vi "DAQ Message Loop.vi"(8 "error in (no error)":errorcluster, 11 "Message Queues":T1) -> (0 "error out":errorcluster)   [LabVIEW 2018, in "DAQ.lvlib"]
doc: "Message loop for handling messages pertaining to the acquisition of data from the hardware."
uses:
  DAQ/DAQ.lvlib
  Main/Main Queue Cluster.ctl
  support/Message Queue/Message Cluster.ctl
  Acquisition State.ctl
  Hardware Configuration.ctl
  Task Cluster.ctl
  controls/Queue and Message Cluster.ctl
  support/Message Queue/Enqueue Message (Single).vi
  support/Message Queue/Message Queue.lvlib
  DAQ/DAQ Write Folder/DAQ/DAQ Write.lvlib
  Acquisition Settings Dialog.vi
  support/Command Log VIs/Command Logging.lvlib
  Report Generation/Report Generation.lvlib
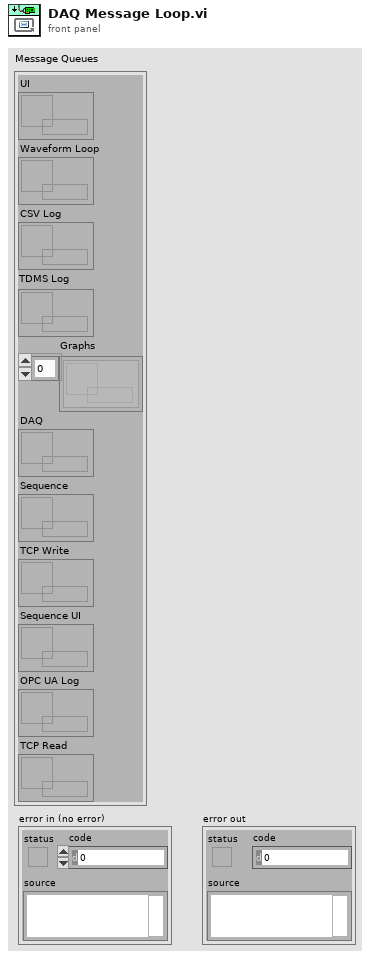
[diagram p1: front panel]
types:
  T1 = typedef "Main Queue Cluster.ctl" = cluster{"UI":refnum<queue>, "Waveform Loop":refnum<queue>, "CSV Log":refnum<queue>, "TDMS Log":refnum<queue>, "Graphs":refnum<queue>[], "DAQ":refnum<queue>, "Sequence":refnum<queue>, "TCP Write":refnum<queue>, "Sequence UI":refnum<queue>, "OPC UA Log":refnum<queue>, "TCP Read":refnum<queue>}
  T2 = typedef "DAQ.lvlib/Hardware Configuration.ctl" = cluster{"Tasks Array":T3[]}
  T3 = typedef "Task Cluster.ctl" = cluster{"DAQmx Task":refnum<k21>, "Read-Write Radio":enum32{"Read", "Write"}}
  T4 = typedef "DAQ.lvlib/DAQ Write.lvlib/Acquisition State.ctl" = enum16{"Idle", "Acquiring"}
  T5 = typedef "Queue and Message Cluster.ctl" = cluster{"return Message Queue":refnum<queue>, "Message":string, "Variant":variant}
  T6 = cluster{"Name":string, "Alarm Time":timestamp}[][]
  T7 = typedef "Message Queue.lvlib/Message Cluster.ctl" = cluster{"Message":string, "Message Data":variant}
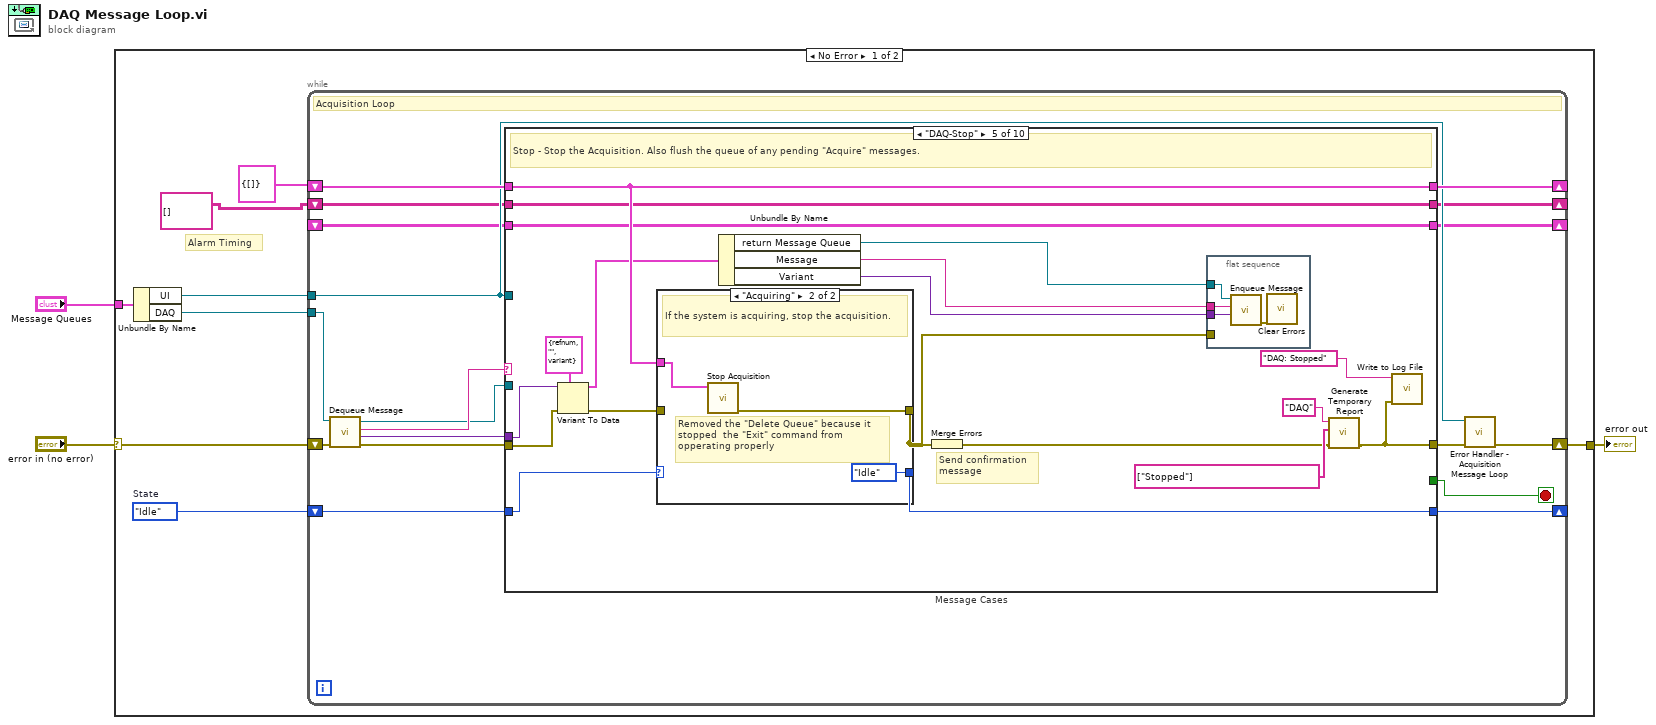
[diagram p0: block diagram]
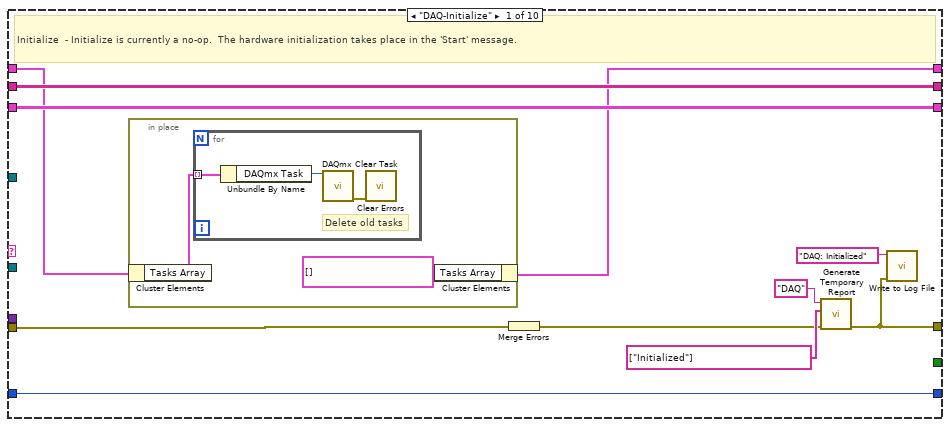
[diagram p2: hidden frame]
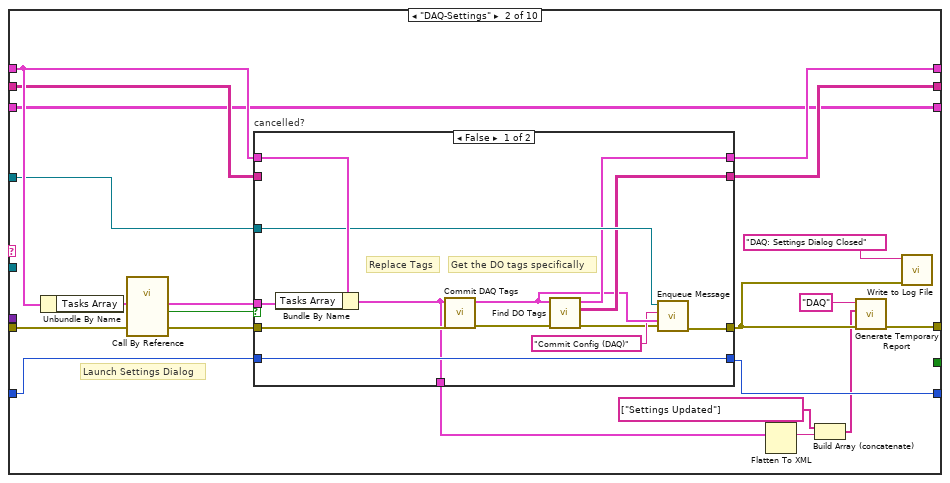
[diagram p3: hidden frame]
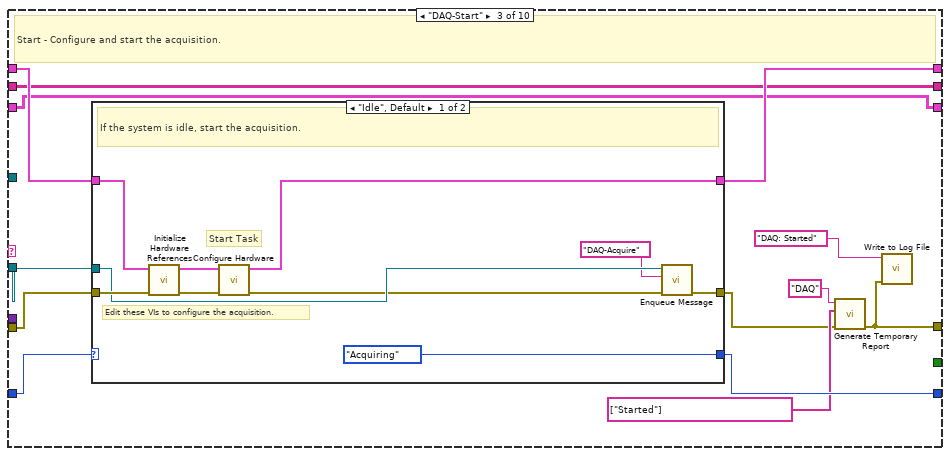
[diagram p5: hidden frame]
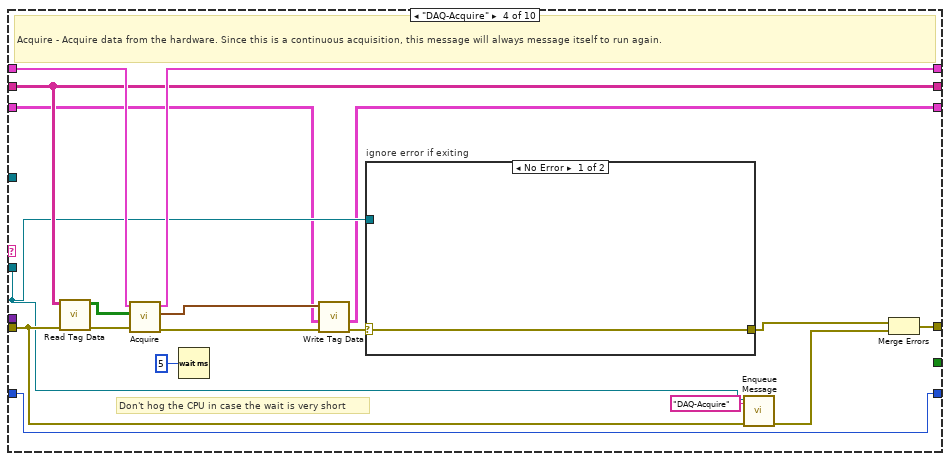
[diagram p7: hidden frame]
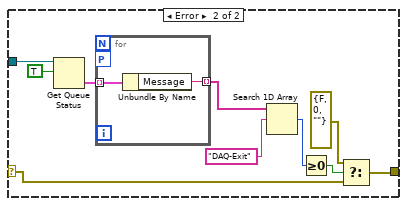
[diagram p8: hidden frame]
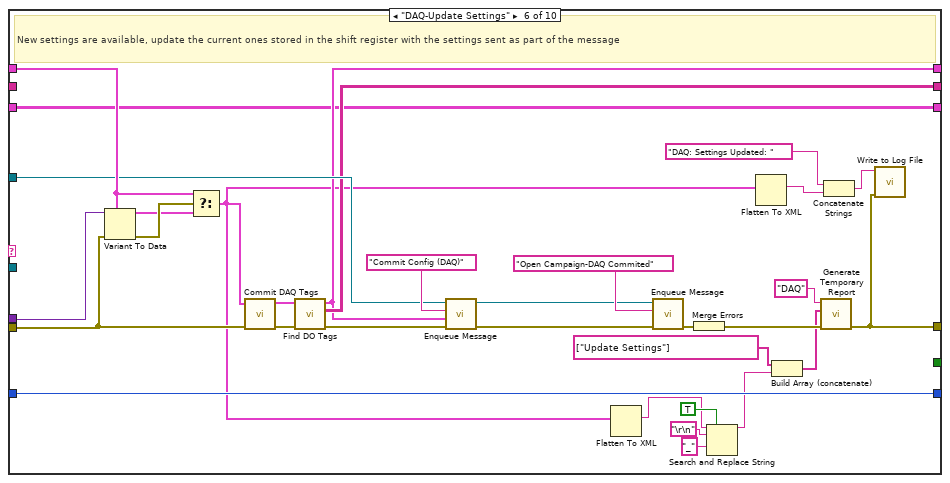
[diagram p10: hidden frame]
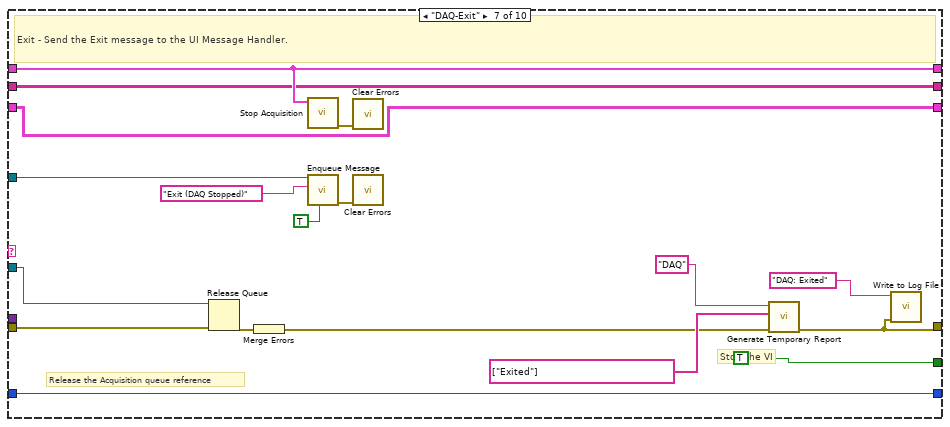
[diagram p11: hidden frame]
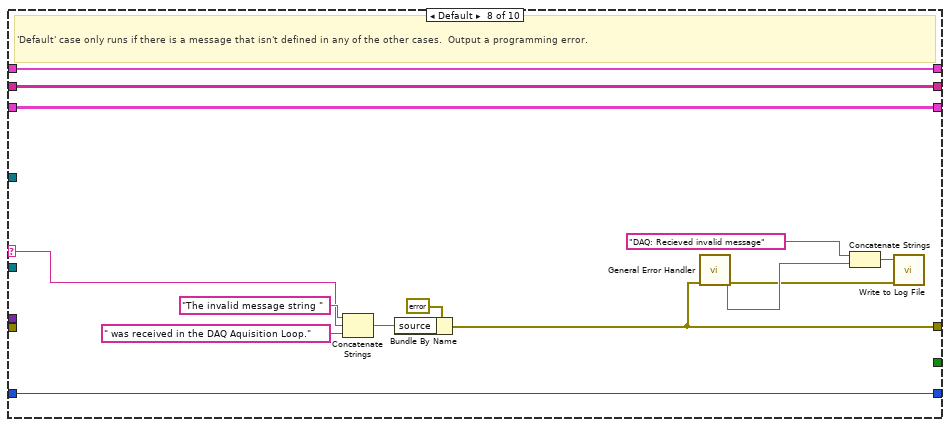
[diagram p12: hidden frame]
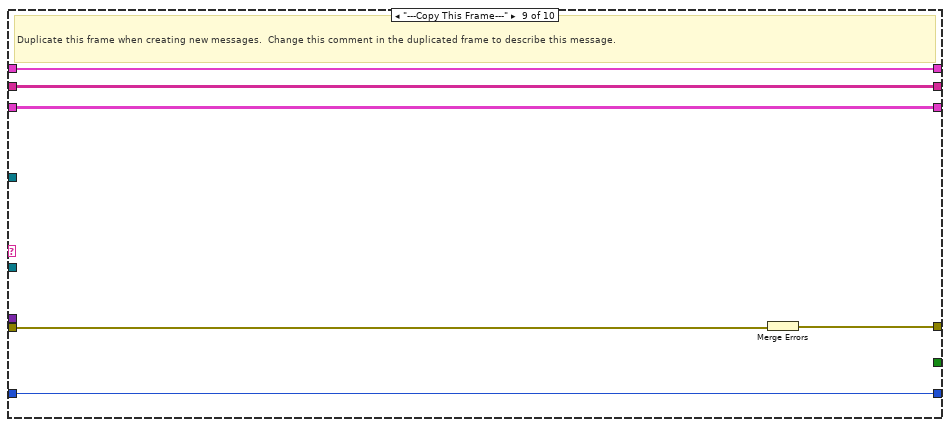
[diagram p13: hidden frame]
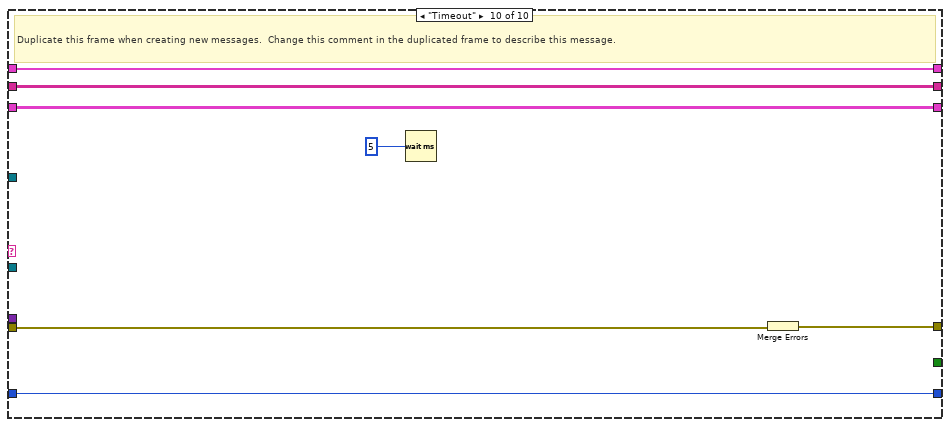
[diagram p14: hidden frame]
diagram:
  n1 = case shown="No Error" "error in (no error)" {
    selector: "error in (no error)" -> [w8 w246]
    tunnel: "Message Queues" -> [w11 _]
    tunnel: [w9 w246] -> w2
    frame No Error {
      w6 = Acquisition_State."Idle"  # State
      # "Alarm Timing"
      n2 = Unbundle By Name(w11) -> ("UI"=w7:refnum<queue>, "DAQ"=w10:refnum<queue>)
      n3 = while {
        tunnel: w10 -> [w23]
        shift-right: [w28] -> _
        shift-left: T2 {"Tasks Array"=[]} ("Data Cluster") -> [w29]
        shift-right: [w21] -> w9
        shift-left: w8 -> [w26]
        tunnel: w7 -> [w20]
        shift-right: [w18] -> _
        shift-left: w6 -> [w19]
        shift-right: [w17] -> _
        shift-left: string[][] [] ("Task D-O Channels") -> [w16]
        shift-right: [w13] -> _
        shift-left: _ -> [w12]
        stop <- w27 stop-if-true
        # "Acquisition Loop"
        n4 = call "Dequeue Message.vi"("error in (no error)"=w26, "Message Queue"=w23) -> ("error out"=w15:errorcluster, "Message Data"=w24:variant, "Message"=w25:string, "dup Message Queue"=w14:refnum<queue>)  [unwired: 6 in]
        n5 = case "Message Cases" shown="\"DAQ-Stop\"" w25 {
          selector: w25 -> [_ _ _ _ _ _ _ w219 _ _]
          tunnel: w15 -> [w40 w65 w95 w119 w153 w195 w216 _ w238 w245]
          tunnel: [w30 w50 w84 w114 w142 w177 w201 w220 w236 w243] -> w22
          tunnel: w29 -> [w35 w63 w96 w126 w159 w197 w212 w232 w237 w244]
          tunnel: [w34 w62 w94 w127 w159 w184 w212 w232 w237 w244] -> w28
          tunnel: [_ _ _ _ _ _ TRUE _ _ _] -> w27
          tunnel: w24 -> [_ _ _ _ w155 w200 _ _ _ _]
          tunnel: w20 -> [_ w59 _ _ _ w190 w217 _ _ _]
          tunnel: w19 -> [w39 w55 w93 w125 w158 w196 w211 w231 w235 w242]
          tunnel: [w39 w54 w92 w125 w157 w196 w211 w231 w235 w242] -> w18
          tunnel: [w38 w58 w91 w116 w147 w185 w208 w230 w234 w241] -> w17
          tunnel: w16 -> [w38 w57 w91 w116 w147 _ w208 w230 w234 w241]
          tunnel: w14 -> [_ _ w90 w115 _ _ w207 _ _ _]
          tunnel: w12 -> [w36 w53 w88 w111 w145 w180 w205 w225 w233 w239]
          tunnel: [w36 w53 w88 w110 w145 w180 w205 w225 w233 w239] -> w13
          frame "DAQ-Initialize" {
            # "Initialize  - Initialize is currently a no-op.  The hardware initialization takes place in the 'Start' message."
            n6 = in-place {
              n7 = in-place-cluster #1(w35) -> ("Tasks Array"=w42:T3[])
              n8 = for {
                tunnel: w42 -> [w45] mode=indexing
                # "Delete old tasks"
                n9 = Unbundle By Name(w45) -> ("DAQmx Task"=w44:refnum<k21>)
                n10 = call <vilib>:"DAQmx Clear Task.vi"("task in"=w44) -> ("error out"=w43:errorcluster)  [unwired: 14 in]
                n11 = call <vilib>:"Clear Errors.vi"("error in (no error)"=w43) -> ()  [unwired: 5 in, 2 out]
              }
              n12 = in-place-cluster #1("Tasks Array"=T3[] [] ("Tasks")) -> (w34:T2)
            }
            n13 = Merge Errors(w40) -> (w31:errorcluster)
            n14 = call "Generate Temporary Report.vi"("error in (no error)"=w31, "Line of Events"=string[] ["Initialized"], "Module Name"="DAQ") -> ("error out"=w30:errorcluster)  [unwired: 8 in]
            n15 = call "Write to Log File.vi"("error in"=w30, "text"="DAQ: Initialized") -> ()  [unwired: 9 in, 1 out]
          }
          frame "DAQ-Settings" {
            # "Launch Settings Dialog"
            n16 = Unbundle By Name(w63) -> ("Tasks Array"=w64:T3[])
            n17 = call-by-ref "?"("error in (no error)"=w65, "Tasks in"=w64) -> ("error out"=w60:errorcluster, "cancelled"=w61:bool, "Tasks out"=w66:T3[])  [unwired: 9 in, 2 out]
            n18 = case "cancelled?" shown="False" w61 {
              tunnel: w66 -> [w75 _]
              tunnel: w63 -> [w79 w80]
              tunnel: [w73 w80] -> w62
              tunnel: w60 -> [w78 w83]
              tunnel: [w77 w83] -> w51
              tunnel: w59 -> [w76 _]
              tunnel: [w74 w82] -> w58
              tunnel: w57 -> [_ w82]
              tunnel: [w70 w81] -> w54
              tunnel: w55 -> [w70 w81]
              tunnel: [w67 w80] -> w47
              frame False {
                # "Get the DO tags specifically"
                # "Replace Tags"
                n19 = Bundle By Name(cluster=w79, "Tasks Array"=w75) -> (w67:T2)
                n20 = call "Commit DAQ Tags.vi"("error in (no error)"=w78, "DAQ State in"=w67) -> ("error out"=w72:errorcluster, "DAQ State out"=w71:T2)  [unwired: 8 in]
                n21 = call "Find DO Tags.vi"("error in (no error)"=w72, "DAQ State in"=w71) -> ("error out"=w68:errorcluster, "Task D-O Channels"=w74:string[][], "DAQ State out"=w73:T2)  [unwired: 7 in]
                n22 = call-poly "Enqueue Message.vi"("error in (no error)"=w68, "Message Data"=w71, "Message"="Commit Config (DAQ)", "Message Queue"=w76) -> ("error out"=w77:errorcluster)  [unwired: 6 in, 1 out]
              }
              frame True {
              }
            }
            n23 = Flatten To XML(anything=w47) -> (xml string=w46:string)
            n24 = Build Array (concatenate)(string[] ["Settings Updated"] ("Line of Events"), w46) -> (w48:string[])
            n25 = call "Generate Temporary Report.vi"("error in (no error)"=w51, "Line of Events"=w48, "Module Name"="DAQ") -> ("error out"=w50:errorcluster)  [unwired: 8 in]
            n26 = call "Write to Log File.vi"("error in"=w51, "text"="DAQ: Settings Dialog Closed") -> ()  [unwired: 9 in, 1 out]
          }
          frame "DAQ-Start" {
            # "Start - Configure and start the acquisition."
            n27 = case shown="\"Idle\", Default" w93 {
              selector: w93 -> [_ w107]
              tunnel: [w99 w109] -> w85
              tunnel: w96 -> [w106 w108]
              tunnel: w95 -> [w101 w109]
              tunnel: w90 -> [w100 _]
              tunnel: [w103 w108] -> w94
              tunnel: [Acquisition_State."Acquiring" ("State") w107] -> w92
              frame "Idle", Default {
                # "Start Task"
                # "Edit these VIs to configure the acquisition."
                # "If the system is idle, start the acquisition."
                n28 = call "Initialize Hardware References.vi"("error in (no error)"=w101, "Hardware Resources in"=w106) -> ("error out"=w105:errorcluster, "Hardware Resources out"=w104:T2)  [unwired: 8 in]
                n29 = call "Configure Hardware.vi"("error in (no error)"=w105, "Hardware Resources in"=w104) -> ("error out"=w97:errorcluster, "Hardware Resources out"=w103:T2)  [unwired: 8 in]
                n30 = call-poly "Enqueue Message.vi"("error in (no error)"=w97, "Message"="DAQ-Acquire", "Message Queue"=w100) -> ("error out"=w99:errorcluster)  [unwired: 7 in, 1 out]
              }
              frame "Acquiring" {
                # "The system is already acquiring. Ignore the \"Start\" message."
              }
            }
            n31 = call "Generate Temporary Report.vi"("error in (no error)"=w85, "Line of Events"=string[] ["Started"], "Module Name"="DAQ") -> ("error out"=w84:errorcluster)  [unwired: 8 in]
            n32 = call "Write to Log File.vi"("error in"=w84, "text"="DAQ: Started") -> ()  [unwired: 9 in, 1 out]
          }
          frame "DAQ-Acquire" {
            # "Don't hog the CPU in case the wait is very short"
            # "Acquire - Acquire data from the hardware. Since this is a continuous acquisition, this message will always message itself to run again."
            n33 = call "Read Tag Data.vi"("error in (no error)"=w119, "Task D-O Channels"=w116) -> ("error out"=w118:errorcluster, "Array"=w120:bool[][])  [unwired: 8 in]
            n34 = call "Acquire.vi"("error in (no error)"=w118, "Digital Write Status"=w120, "Hardware Resources in"=w126) -> ("error out"=w113:errorcluster, "data"=w124:waveform(dbl)[], "Hardware Resources out"=w127:T2)  [unwired: 6 in]
            n35 = Wait (ms)(milliseconds to wait=u32 5) -> ()  [unwired: 1 out]
            n36 = call "Write Tag Data.vi"("error in (no error)"=w113, "Alarms Time Array"=w111, "data"=w124) -> ("error out"=w112:errorcluster, "Alarm Time Array"=w110:T6)  [unwired: 5 in, 2 out]
            n37 = case "ignore error if exiting" shown="No Error" w112 {
              selector: w112 -> [w128 w131]
              tunnel: w115 -> [_ w138]
              tunnel: [w128 w130] -> w122
              frame No Error {
              }
              frame Error {
                n38 = Get Queue Status(queue=w138, return elements? (F)=TRUE) -> (elements=w135:T7[])  [unwired: 1 in, 7 out]
                n39 = for {
                  tunnel: w135 -> [w140] mode=indexing
                  tunnel: [w139] -> w134 mode=indexing
                  workers-P: _ -> [_]
                  n40 = Unbundle By Name(w140) -> ("Message"=w139:string)
                }
                n41 = Search 1D Array(1D array=w134, element="DAQ-Exit") -> (index of element=w133:i32)  [unwired: 1 in]
                n42 = Greater Or Equal To 0?(x=w133) -> (x >= 0?=w132:bool)
                n43 = Select(t=errorcluster {"status"=FALSE, "code"=0, "source"=""}, s=w132, f=w131) -> (s? t:f=w130:errorcluster)
              }
            }
            n44 = call-poly "Enqueue Message.vi"("error in (no error)"=w119, "Message"="DAQ-Acquire", "Message Queue"=w115) -> ("error out"=w121:errorcluster)  [unwired: 7 in, 1 out]
            n45 = Merge Errors(w122, w121) -> (w114:errorcluster)
          }
          frame "DAQ-Stop" {
            # "Send confirmation\nmessage"
            # "Stop - Stop the Acquisition. Also flush the queue of any pending \"Acquire\" messages."
            n46 = Variant To Data(error in=w153, type=T5 {"return Message Queue"=refnum, "Message"="", "Variant"=variant} ("Queue and Message"), Variant=w155) -> (data=w152:T5, error out=w154:errorcluster)
            n47 = case shown="\"Acquiring\"" w158 {
              selector: w158 -> [w165 _]
              tunnel: w154 -> [w164 _]
              tunnel: w159 -> [_ w168]
              tunnel: [w165 Acquisition_State."Idle" ("State")] -> w157
              tunnel: [w164 w166] -> w148
              frame "Idle", Default {
                # "The system is already idle. Ignore the \"Stop\" message."
              }
              frame "Acquiring" {
                # "Removed the \"Delete Queue\" because it\nstopped  the \"Exit\" command from \nopperating properly"
                # "If the system is acquiring, stop the acquisition."
                n48 = call "Stop Acquisition.vi"("Hardware Resources in"=w168) -> ("error out"=w166:errorcluster)  [unwired: 10 in]
              }
            }
            n49 = Unbundle By Name(w152) -> ("return Message Queue"=w151:refnum<queue>, "Message"=w150:string, "Variant"=w149:variant)
            n50 = Merge Errors(w148) -> (w141:errorcluster)
            n51 = flat-sequence {
              tunnel: w151 -> [w163]
              tunnel: w150 -> [w162]
              tunnel: w149 -> [w161]
              tunnel: w148 -> [_]
              frame #0 {
                n52 = call-poly "Enqueue Message.vi"("Message Data"=w161, "Message"=w162, "Message Queue"=w163) -> ("error out"=w160:errorcluster)  [unwired: 7 in, 1 out]
                n53 = call <vilib>:"Clear Errors.vi"("error in (no error)"=w160) -> ()  [unwired: 5 in, 2 out]
              }
            }
            n54 = call "Generate Temporary Report.vi"("error in (no error)"=w141, "Line of Events"=string[] ["Stopped"], "Module Name"="DAQ") -> ("error out"=w142:errorcluster)  [unwired: 8 in]
            n55 = call "Write to Log File.vi"("error in"=w142, "text"="DAQ: Stopped") -> ()  [unwired: 9 in, 1 out]
          }
          frame "DAQ-Update Settings" {
            # "New settings are available, update the current ones stored in the shift register with the settings sent as part of the message"
            n56 = Variant To Data(error in=w195, type=w197, Variant=w200) -> (data=w198:T2, error out=w199:errorcluster)
            n57 = Select(t=w197, s=w199, f=w198) -> (s? t:f=w175:T2)
            n58 = call "Commit DAQ Tags.vi"("error in (no error)"=w195, "DAQ State in"=w175) -> ("error out"=w192:errorcluster, "DAQ State out"=w186:T2)  [unwired: 8 in]
            n59 = call "Find DO Tags.vi"("error in (no error)"=w192, "DAQ State in"=w186) -> ("error out"=w189:errorcluster, "Task D-O Channels"=w185:string[][], "DAQ State out"=w184:T2)  [unwired: 7 in]
            n60 = call-poly "Enqueue Message.vi"("error in (no error)"=w189, "Message Data"=w184, "Message"="Commit Config (DAQ)", "Message Queue"=w190) -> ("error out"=w188:errorcluster, "dup Message Queue"=w187:refnum<queue>)  [unwired: 6 in]
            n61 = Flatten To XML(anything=w175) -> (xml string=w170:string)
            n62 = call-poly "Enqueue Message.vi"("error in (no error)"=w188, "Message"="Open Campaign-DAQ Commited", "Message Queue"=w187) -> ("error out"=w194:errorcluster)  [unwired: 7 in, 1 out]
            n63 = Merge Errors(w194) -> (w178:errorcluster)
            n64 = Search and Replace String(replace all?=TRUE ("replace all? (F)"), input string=w170, search string="\r\n", replace string="_" ("replace string (\"\")")) -> (result string=w169:string)  [unwired: 4 in, 3 out]
            n65 = Flatten To XML(anything=w175) -> (xml string=w181:string)
            n66 = Build Array (concatenate)(string[] ["Update Settings"] ("Line of Events"), w169) -> (w174:string[])
            n67 = call "Generate Temporary Report.vi"("error in (no error)"=w178, "Line of Events"=w174, "Module Name"="DAQ") -> ("error out"=w177:errorcluster)  [unwired: 8 in]
            n68 = Concatenate Strings("DAQ: Settings Updated: " ("text"), w181) -> (w182:string)
            n69 = call "Write to Log File.vi"("error in"=w177, "text"=w182) -> ()  [unwired: 9 in, 1 out]
          }
          frame "DAQ-Exit" {
            # "Release the Acquisition queue reference"
            # "Stop the VI"
            # "Exit - Send the Exit message to the UI Message Handler."
            n70 = Release Queue(queue=w207, error in (no error)=w216) -> (error out=w213:errorcluster)  [unwired: 1 in, 2 out]
            n71 = Merge Errors(w213) -> (w202:errorcluster)
            n72 = call "Stop Acquisition.vi"("Hardware Resources in"=w212) -> ("error out"=w210:errorcluster)  [unwired: 10 in]
            n73 = call-poly "Enqueue Message.vi"("Priority Message? (F)"=TRUE, "Message"="Exit (DAQ Stopped)", "Message Queue"=w217) -> ("error out"=w209:errorcluster)  [unwired: 7 in, 1 out]
            n74 = call <vilib>:"Clear Errors.vi"("error in (no error)"=w210) -> ()  [unwired: 5 in, 2 out]
            n75 = call <vilib>:"Clear Errors.vi"("error in (no error)"=w209) -> ()  [unwired: 5 in, 2 out]
            n76 = call "Generate Temporary Report.vi"("error in (no error)"=w202, "Line of Events"=string[] ["Exited"], "Module Name"="DAQ") -> ("error out"=w201:errorcluster)  [unwired: 8 in]
            n77 = call "Write to Log File.vi"("error in"=w201, "text"="DAQ: Exited") -> ()  [unwired: 9 in, 1 out]
          }
          frame Default {
            # "'Default' case only runs if there is a message that isn't defined in any of the other cases.  Output a programming error."
            n78 = Concatenate Strings("The invalid message string " ("string"), w219, " was received in the DAQ Aquisition Loop." ("string")) -> (w221:string)
            n79 = Bundle By Name(cluster=errorcluster {"status"=TRUE, "code"=1, "source"=""} ("error constant"), "source"=w221) -> (w220:errorcluster)
            n80 = call <vilib>:"General Error Handler.vi"("error in (no error)"=w220) -> ("message"=w227:string, "error out"=w226:errorcluster)  [unwired: 10 in, 3 out]
            n81 = Concatenate Strings("DAQ: Recieved invalid message" ("text"), w227) -> (w229:string)
            n82 = call "Write to Log File.vi"("error in"=w226, "text"=w229) -> ()  [unwired: 9 in, 1 out]
          }
          frame "---Copy This Frame---" {
            # "Duplicate this frame when creating new messages.  Change this comment in the duplicated frame to describe this message."
            n83 = Merge Errors(w238) -> (w236:errorcluster)
          }
          frame "Timeout" {
            # "Duplicate this frame when creating new messages.  Change this comment in the duplicated frame to describe this message."
            n84 = Wait (ms)(milliseconds to wait=u32 5) -> ()  [unwired: 1 out]
            n85 = Merge Errors(w245) -> (w243:errorcluster)
          }
        }
        n86 = call "Error Handler - Acquisition Message Loop.vi"("error in (no error)"=w22, "Message Queue"=w20) -> ("dup error in"=w21:errorcluster)  [unwired: 8 in, 1 out]
      }
    }
    frame Error {
    }
  }
  "error out" <- w2
